vi "Wait miliseconds.vi"(8 "error in (no error)":errorcluster, 11 "milliseconds to wait":u32=10) -> (0 "error out":errorcluster, 3 "millisecond timer value":u32)   [LabVIEW 2015]
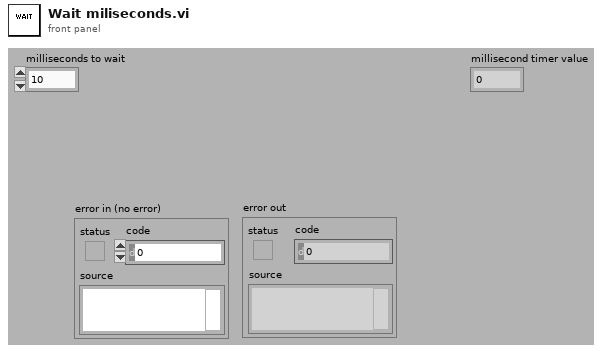
[diagram p1: front panel]
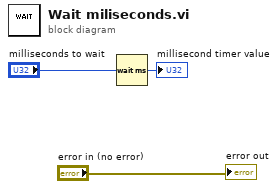
[diagram p0: block diagram]
diagram:
  n1 = Wait (ms)(milliseconds to wait="milliseconds to wait") -> (millisecond timer value=→"millisecond timer value":u32)
  "error out" <- "error in (no error)"
